vi "SENS_IF_FILT_SAMP_PER_CAT.vi"(0 "VISA IN":refnum<visa-resource-name>, 5 "error in":errorcluster, 7 "Channel":i32) -> (14 "VISA Out":refnum<visa-resource-name>, 19 "error out":errorcluster)   [LabVIEW 2018, in "PNA-X.lvlib"]
doc: "SENSe<cnum>:IF:FILTer:SAMPle:PERiod:CATalog? \n(Read-Only) Returns the list of allowed IF filter sample periods for this instrument. Critical Note: \nParameters \n<cnum> Existing channel number to manipulate. If unspecified, <cnum> is set to 1. \nExamples SENS:IF:FILT:SAMP:PER:CAT? \nsense2:if:filter:sample:period:catalog? \nQuery Syntax SENS:IF:FILTer:SAMPle:PERiod:CATalog? \nReturn Type String \nDefault AUTO \n1749"
uses:
  PNA-X.lvlib
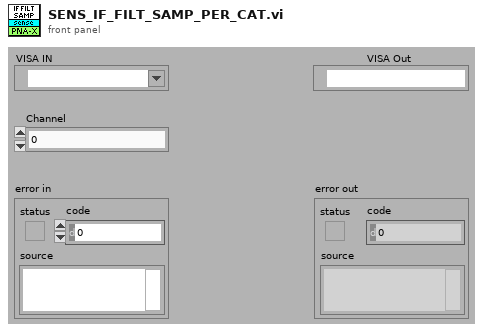
[diagram p1: front panel]
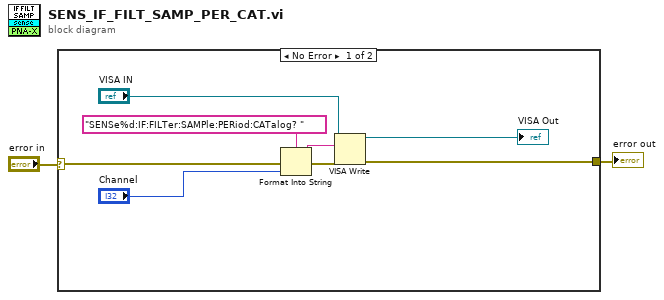
[diagram p0: block diagram]
diagram:
  n1 = case shown="No Error" "error in" {
    selector: "error in" -> [w10 w11]
    tunnel: [w4 w11] -> w1
    frame No Error {
      n2 = Format Into String(format string="SENSe%d:IF:FILTer:SAMPle:PERiod:CATalog? " ("Cmdline"), error in=w10, "Channel") -> (resulting string=w8:string, error out=w9:errorcluster)  [unwired: 1 in]
      n3 = VISA Write(VISA resource name="VISA IN", write buffer=w8, error in (no error)=w9) -> (VISA resource name out=→"VISA Out":refnum<visa-resource-name>, error out=w4:errorcluster)  [unwired: 1 out]
    }
    frame Error {
    }
  }
  "error out" <- w1
